vi "GetAllPathes.vi"(9 "EndPoistion":cluster{"x":i32, "y":i32}, 10 "CurrentPoistion":cluster{"x":i32, "y":i32}, 11 "PathIn":cluster{"dX":i32, "dY":i32}[](array[cluster])) -> (2 "EndFound":bool, 3 "PathOut":cluster{"dX":i32, "dY":i32}[][](array[cluster]))   [LabVIEW 2020, in "2021_15.lvclass"]
uses:
  2021_15.lvclass
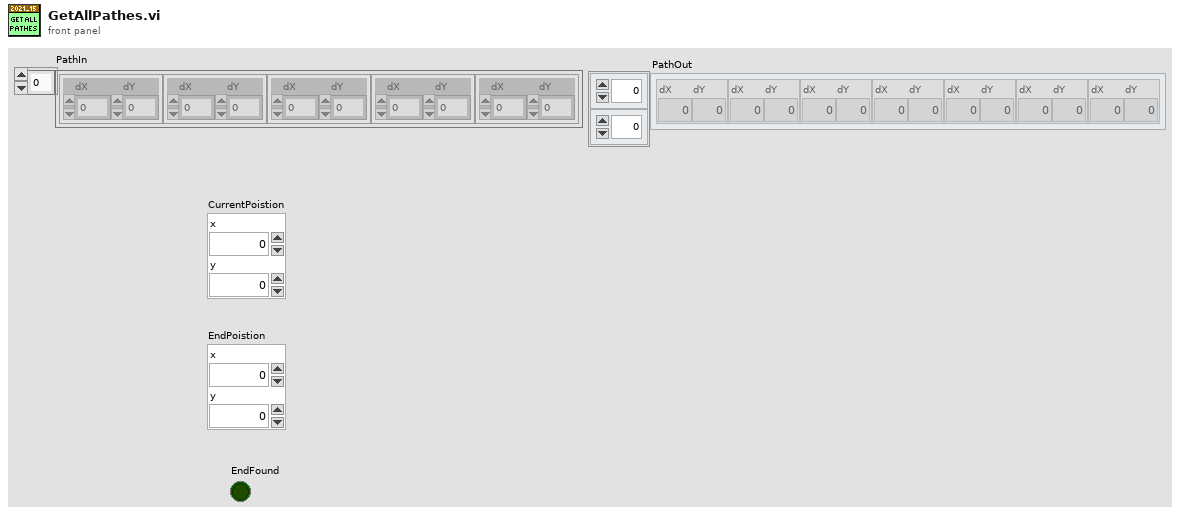
[diagram p1: front panel]
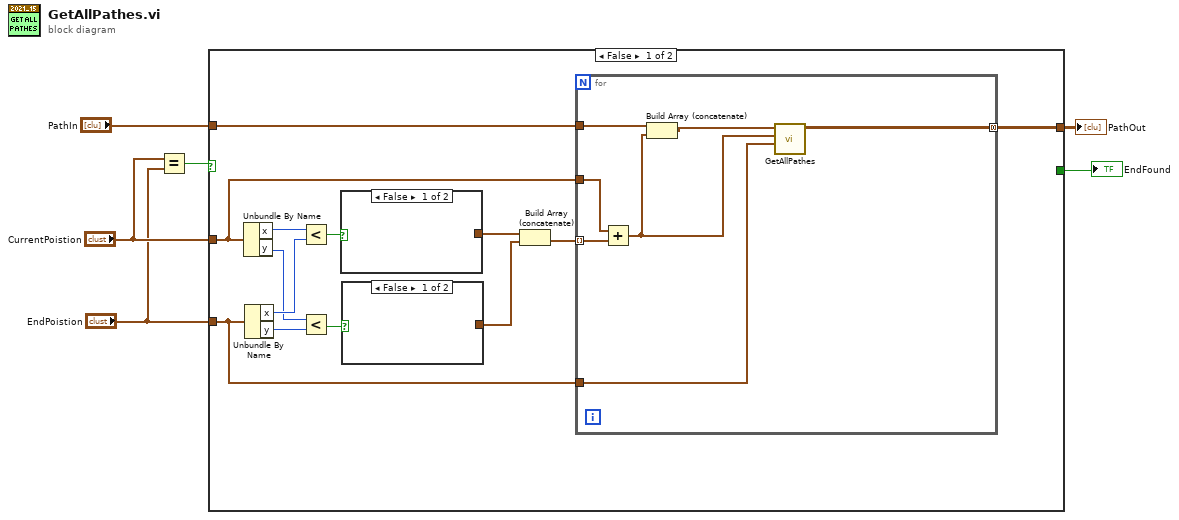
[diagram p0: block diagram]
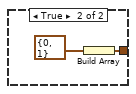
[diagram p2: hidden frame]
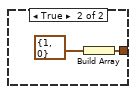
[diagram p3: hidden frame]
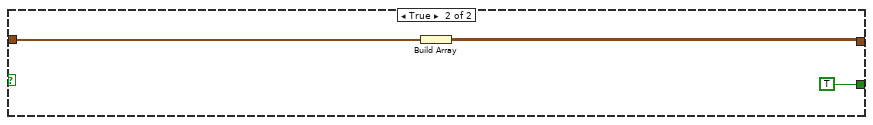
[diagram p4: hidden frame]
diagram:
  n1 = Equal?(x="CurrentPoistion", y="EndPoistion") -> (x = y?=w4:bool)
  n2 = case shown="False" w4 {
    tunnel: "CurrentPoistion" -> [w10 _]
    tunnel: "EndPoistion" -> [w9 _]
    tunnel: "PathIn" -> [w8 w32]
    tunnel: [_ TRUE] -> w2
    tunnel: [w7 w31] -> w1
    frame False {
      n3 = Unbundle By Name(w10) -> ("x"=w19:i32, "y"=w16:i32)
      n4 = Unbundle By Name(w9) -> ("x"=w18:i32, "y"=w15:i32)
      n5 = Less?(x=w19, y=w18) -> (x < y?=w17:bool)
      n6 = Less?(x=w16, y=w15) -> (x < y?=w14:bool)
      n7 = case shown="False" w17 {
        tunnel: [_ w29] -> w13
        frame False {
        }
        frame True {
          n8 = Build Array(cluster{"dX":i32, "dY":i32} {"dX"=1, "dY"=0} ("Cluster")) -> (w29:cluster{"dX":i32, "dY":i32}[])
        }
      }
      n9 = case shown="False" w14 {
        tunnel: [_ w27] -> w12
        frame False {
        }
        frame True {
          n10 = Build Array(cluster{"dX":i32, "dY":i32} {"dX"=0, "dY"=1} ("Cluster")) -> (w27:cluster{"dX":i32, "dY":i32}[])
        }
      }
      n11 = Build Array (concatenate)(w13, w12) -> (w11:cluster{"dX":i32, "dY":i32}[])
      n12 = for {
        tunnel: w10 -> [w26]
        tunnel: w11 -> [w25] mode=indexing
        tunnel: w9 -> [w24]
        tunnel: w8 -> [w23]
        tunnel: [w20] -> w7 mode=concatenating
        n13 = Add(x=w26, y=w25) -> (x+y=w22:cluster{i32, i32})
        n14 = Build Array (concatenate)(w23, w22) -> (w21:cluster{"dX":i32, "dY":i32}[])
        n15 = call "GetAllPathes.vi"("EndPoistion"=w24, "CurrentPoistion"=w22, "PathIn"=w21) -> ("PathOut"=w20:cluster{"dX":i32, "dY":i32}[][])  [unwired: 7 in, 1 out]
      }
    }
    frame True {
      n16 = Build Array(w32) -> (w31:cluster{"dX":i32, "dY":i32}[][])
    }
  }
  "EndFound" <- w2
  "PathOut" <- w1
